vi "Start.vi"(8 "error in (no error)":errorcluster, 11 "Server in":refnum<class "Server.lvclass">) -> (0 "error out":errorcluster, 3 "Server out":refnum<class "Server.lvclass">)   [LabVIEW 2020, in "Server.lvlib" / "Server.lvclass"]
doc: "Start the server. This will make the added PVs available via PVAccess."
uses:
  Server.lvclass
  Server.lvclass/Server.ctl
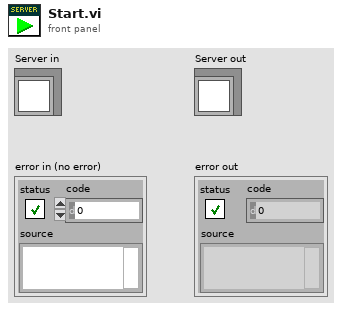
[diagram p1: front panel]
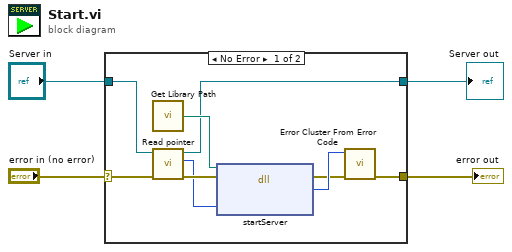
[diagram p0: block diagram]
diagram:
  n1 = case shown="No Error" "error in (no error)" {
    selector: "error in (no error)" -> [w9 w15]
    tunnel: [w11 w15] -> w2
    tunnel: [w5 w14] -> w3
    tunnel: "Server in" -> [w6 w14]
    frame No Error {
      n2 = call "Get Library Path.vi"() -> ("Path"=w10:path)  [unwired: 1 in]
      n3 = call "Read pointer.vi"("error in (no error)"=w9, "Server in"=w6) -> ("error out"=w8:errorcluster, "server pointer"=w7:i64, "Server out"=w5:refnum<class "Server.lvclass">)  [unwired: 7 in]
      n4 = dll-call lib="?" fn="startServer"(path in=w10, error in=w8, "server"=w7) -> (error out=w12:errorcluster, "ret code"=w13:i32)  [unwired: 2 in, 1 out]
      n5 = call <vilib>:"Error Cluster From Error Code.vi"("error in (no error)"=w12, "error code (0)"=w13) -> ("error out"=w11:errorcluster)  [unwired: 7 in]
    }
    frame Error {
    }
  }
  "error out" <- w2
  "Server out" <- w3
